vi "CAN write.vi"(4 "error in (no error)":errorcluster, 5 "Data":u8[](array[numeric]), 6 "COB id":i32, 7 "CANopen in":refnum<class "CANopen.lvclass">) -> (0 "error out":errorcluster, 3 "CANopen out":refnum<class "CANopen.lvclass">)   [LabVIEW 2024, in "canopen.lvlib" / "CANopen.lvclass"]
doc: "Sends a bunch of data to a specific COB-ID."
uses:
  CANopen.lvclass
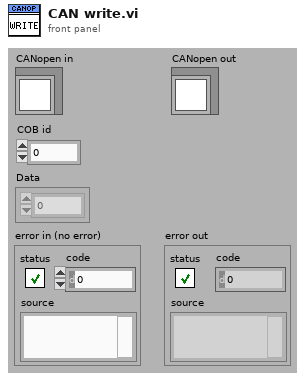
[diagram p1: front panel]
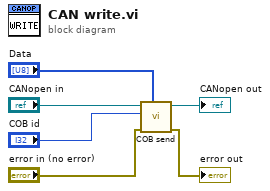
[diagram p0: block diagram]
diagram:
  n1 = call "COB send.vi"("Data"="Data", "error in"="error in (no error)", "COB id"="COB id", "CANopen in"="CANopen in") -> ("error out"=→"error out":errorcluster, "CANopen out"=→"CANopen out":refnum<class "CANopen.lvclass">)  [unwired: 1 in, 2 out]
